vi "Dimensions.vi"(11 "Image In":T1) -> (0 "width":i32, 1 "height":i32, 3 "Image out":T1)   [LabVIEW 2019]
uses:
  <vilib>/picture/picture.llb/imagedata.ctl
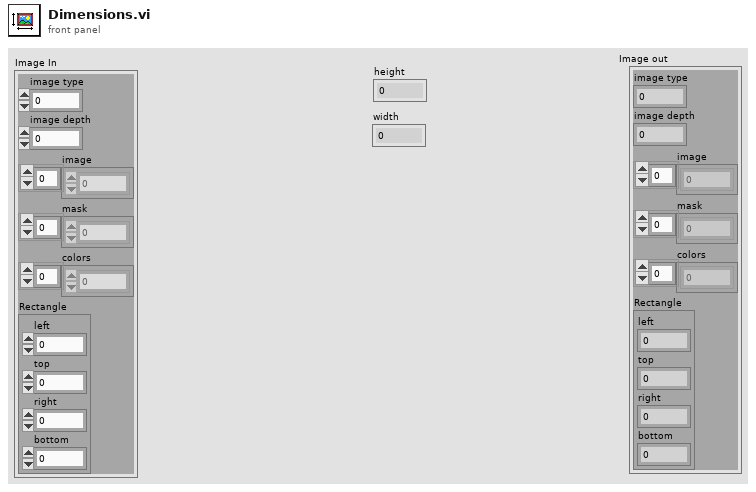
[diagram p1: front panel]
types:
  T1 = typedef "imagedata.ctl" = cluster{"image type":i32, "image depth":i32, "image":u8[], "mask":u8[], "colors":u32[], "Rectangle":cluster{"left":i16, "top":i16, "right":i16, "bottom":i16}}
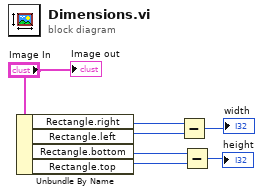
[diagram p0: block diagram]
diagram:
  n1 = Unbundle By Name("Image In") -> ("Rectangle.right"=w6:i16, "Rectangle.left"=w5:i16, "Rectangle.bottom"=w3:i16, "Rectangle.top"=w2:i16)
  n2 = Subtract(x=w6, y=w5) -> (x-y=→"width":i16)
  n3 = Subtract(x=w3, y=w2) -> (x-y=→"height":i16)
  "Image out" <- "Image In"
